vi "Controls to Commands 2016.vi"(10 "Pilot-CoPilot Controls":T3) -> (2 "Robot Commands":T1)   [LabVIEW 2015]
uses:
  Robot Control Outputs 2016.ctl
  Robot Commands 2016.ctl
  Load SS/Roller State.ctl
  Global Variables/Temp Variables.vi
  Global Variables/Settings.vi
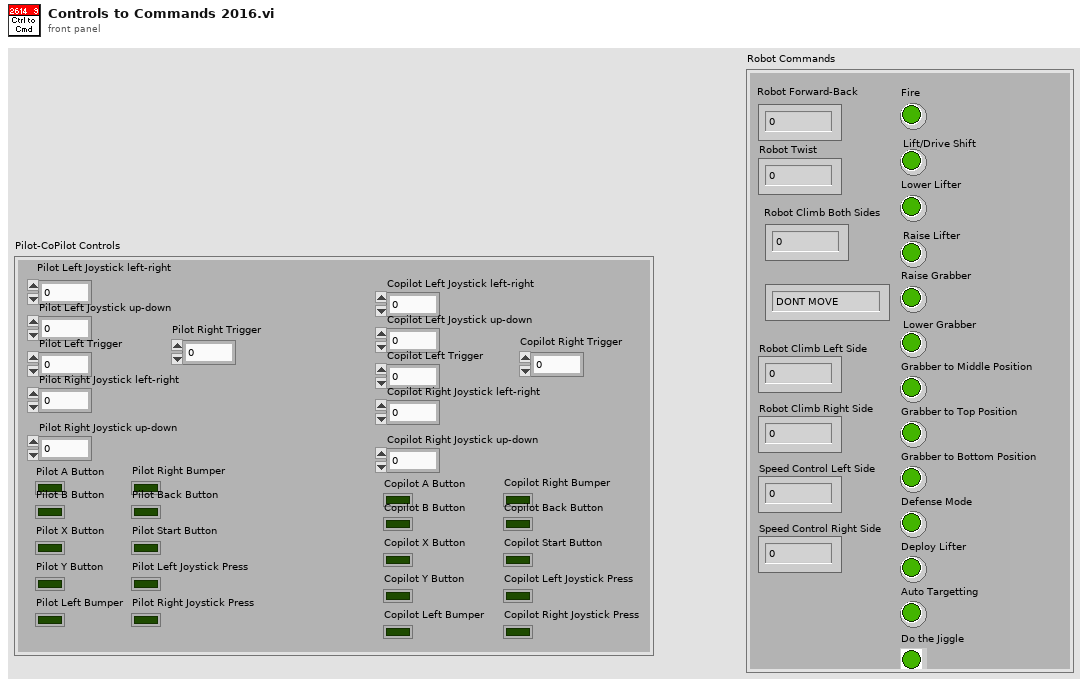
[diagram p1: front panel]
types:
  T1 = typedef "Robot Commands 2016.ctl" = cluster{"Robot Forward-Back":dbl, "Robot Twist":dbl, "Fire":bool, "Lift/Drive Shift":bool, "Raise Lifter":bool, "Raise Grabber":bool, "Lower Grabber":bool, "Roller":T2, "Robot Climb Both Sides":dbl, "Grabber to Middle Position":bool, "Grabber to Top Position":bool, "Grabber to Bottom Position":bool, "Robot Climb Left Side":dbl, "Robot Climb Right Side":dbl, "Speed Control Left Side":dbl, "Speed Control Right Side":dbl, "Lower Lifter":bool, "Defense Mode":bool, "Deploy Lifter":bool, "Auto Targetting":bool, "Do the Jiggle":bool}
  T2 = typedef "Roller State.ctl" = enum16{"DONT MOVE", "Intake", "Outtake"}
  T3 = typedef "Robot Control Outputs 2016.ctl" = cluster{"Pilot Left Joystick left-right":dbl, "Pilot Left Joystick up-down":dbl, "Pilot A Button":bool, "Pilot B Button":bool, "Pilot X Button":bool, "Pilot Y Button":bool, "Pilot Left Bumper":bool, "Pilot Right Bumper":bool, "Pilot Back Button":bool, "Pilot Start Button":bool, "Pilot Left Joystick Press":bool, "Pilot Right Joystick Press":bool, "Pilot Left Trigger":dbl, "Pilot Right Joystick left-right":dbl, "Pilot Right Joystick up-down":dbl, "Pilot Right Trigger":dbl, "Copilot Left Joystick left-right":dbl, "Copilot Left Joystick up-down":dbl, "Copilot A Button":bool, "Copilot B Button":bool, "Copilot X Button":bool, "Copilot Y Button":bool, "Copilot Left Bumper":bool, "Copilot Right Bumper":bool, "Copilot Back Button":bool, "Copilot Start Button":bool, "Copilot Left Joystick Press":bool, "Copilot Right Joystick Press":bool, "Copilot Left Trigger":dbl, "Copilot Right Joystick left-right":dbl, "Copilot Right Joystick up-down":dbl, "Copilot Right Trigger":dbl}
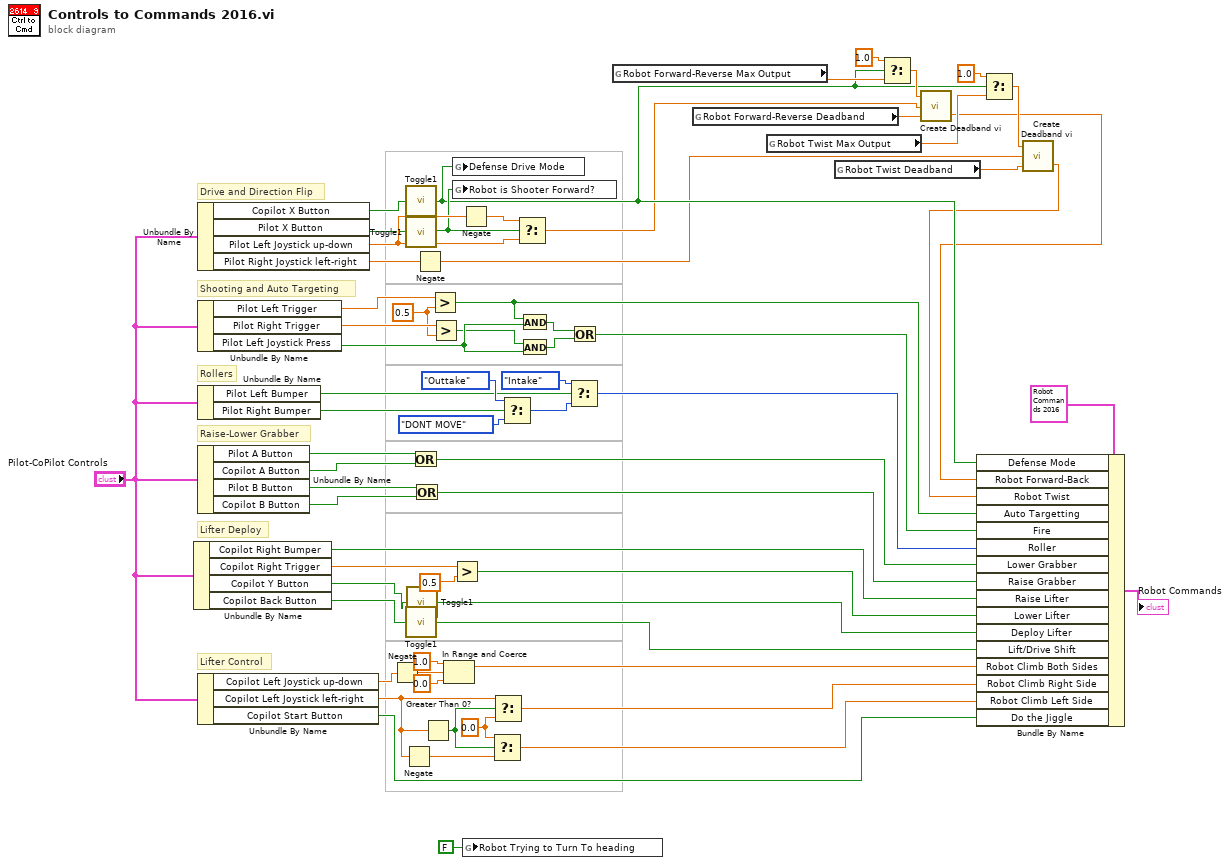
[diagram p0: block diagram]
diagram:
  w28 = 0.0 ("t")
  w63 = 0.5 ("y")
  # "Lifter Control"
  # "Lifter Deploy"
  # "Raise-Lower Grabber"
  # "Rollers"
  # "Shooting and Auto Targeting"
  # "Drive and Direction Flip"
  n1 = Unbundle By Name("Pilot-CoPilot Controls") -> ("Copilot Right Bumper"=w34:bool, "Copilot Right Trigger"=w32:dbl, "Copilot Y Button"=w17:bool, "Copilot Back Button"=w22:bool)
  n2 = Unbundle By Name("Pilot-CoPilot Controls") -> ("Copilot X Button"=w21:bool, "Pilot X Button"=w46:bool, "Pilot Left Joystick up-down"=w48:dbl, "Pilot Right Joystick left-right"=w49:dbl)
  n3 = Unbundle By Name("Pilot-CoPilot Controls") -> ("Pilot Left Trigger"=w64:dbl, "Pilot Right Trigger"=w65:dbl, "Pilot Left Joystick Press"=w61:bool)
  n4 = Unbundle By Name("Pilot-CoPilot Controls") -> ("Pilot Left Bumper"=w52:bool, "Pilot Right Bumper"=w51:bool)
  n5 = Unbundle By Name("Pilot-CoPilot Controls") -> ("Pilot A Button"=w44:bool, "Copilot A Button"=w43:bool, "Pilot B Button"=w42:bool, "Copilot B Button"=w41:bool)
  n6 = Unbundle By Name("Pilot-CoPilot Controls") -> ("Copilot Left Joystick up-down"=w30:dbl, "Copilot Left Joystick left-right"=w25:dbl, "Copilot Start Button"=w15:bool)
  n7 = Negate(x=w30) -> (-x=w35:dbl)
  n8 = Negate(x=w25) -> (-x=w26:dbl)
  n9 = call "Toggle1.vi"("Boolean"=w21) -> ("Driver Switch 2"=w6:bool)
  n10 = call "Toggle1.vi"("Boolean"=w46) -> ("Driver Switch 2"=w45:bool)
  n11 = call "Toggle1.vi"("Boolean"=w22) -> ("Driver Switch 2"=w18:bool)
  n12 = call "Toggle1.vi"("Boolean"=w17) -> ("Driver Switch 2"=w16:bool)
  n13 = Or(x=w44, y=w43) -> (x .or. y?=w40:bool)
  n14 = Or(x=w42, y=w41) -> (x .or. y?=w39:bool)
  n15 = Negate(x=w49) -> (-x=w4:dbl)
  n16 = Greater Than 0?(x=w25) -> (x > 0?=w27:bool)
  n17 = Greater?(x=w64, y=w63) -> (0:w62:bool)
  n18 = Greater?(x=w65, y=w63) -> (0:w60:bool)
  n19 = In Range and Coerce(upper limit=1.0 ("lower limit"), x=w35, lower limit=0.0) -> (coerced(x)=w29:dbl)  [unwired: 1 out]
  n20 = Greater?(x=w32, y=0.5) -> (0:w31:bool)
  n21 = global write "Temp Variables.vi" "Defense Drive Mode"(w6) -> ()
  n22 = global write "Temp Variables.vi" "Robot is Shooter Forward?"(w45) -> ()
  n23 = Negate(x=w48) -> (-x=w47:dbl)
  n24 = global write "Temp Variables.vi" "Robot Trying to Turn To heading"(FALSE ("Robot Trying to Turn To heading")) -> ()
  n25 = Select(t=w28, s=w27, f=w26) -> (s? t:f=w23:dbl)
  n26 = Select(t=w25, s=w27, f=w28) -> (s? t:f=w24:dbl)
  n27 = Select(t=Roller_State."Outtake" ("Roller State"), s=w51, f=Roller_State."DONT MOVE" ("Roller State")) -> (s? t:f=w56:T2)
  n28 = Select(t=w47, s=w45, f=w48) -> (s? t:f=w5:dbl)
  n29 = And(x=w62, y=w61) -> (x .and. y?=w58:bool)
  n30 = And(x=w60, y=w61) -> (x .and. y?=w59:bool)
  n31 = Select(t=Roller_State."Intake" ("Roller State"), s=w52, f=w56) -> (s? t:f=w50:T2)
  n32 = Or(x=w58, y=w59) -> (x .or. y?=w57:bool)
  n33 = global read "Settings.vi" "Robot Forward-Reverse Max Output"() -> (w11:dbl)
  n34 = global read "Settings.vi" "Robot Forward-Reverse Deadband"() -> (w13:dbl)
  n35 = global read "Settings.vi" "Robot Twist Max Output"() -> (w8:dbl)
  n36 = global read "Settings.vi" "Robot Twist Deadband"() -> (w14:dbl)
  n37 = Select(t=1.0, s=w6, f=w11) -> (s? t:f=w12:dbl)
  n38 = call "Create Deadband vi.vi"("Input Deadband"=w13, "Input"=w5, "Output Upper Limit"=w12) -> ("Output"=w3:dbl)  [unwired: 1 in]
  n39 = Select(t=1.0, s=w6, f=w8) -> (s? t:f=w9:dbl)
  n40 = call "Create Deadband vi.vi"("Input Deadband"=w14, "Input"=w4, "Output Upper Limit"=w9) -> ("Output"=w2:dbl)  [unwired: 1 in]
  n41 = Bundle By Name(cluster=T1 {"Robot Forward-Back"=0.0, "Robot Twist"=0.0, "Fire"=FALSE, "Lift/Drive Shift"=FALSE, "Raise Lifter"=FALSE, "Raise Grabber"=FALSE, "Lower Grabber"=FALSE, "Roller"=enum."DONT MOVE", "Robot Climb Both Sides"=0.0, "Grabber to Middle Position"=FALSE, "Grabber to Top Position"=FALSE, "Grabber to Bottom Position"=FALSE, "Robot Climb Left Side"=0.0, "Robot Climb Right Side"=0.0, "Speed Control Left Side"=0.0, "Speed Control Right Side"=0.0, "Lower Lifter"=FALSE, "Defense Mode"=FALSE, "Deploy Lifter"=FALSE, "Auto Targetting"=FALSE, "Do the Jiggle"=FALSE} ("Robot Commands"), "Defense Mode"=w6, "Robot Forward-Back"=w3, "Robot Twist"=w2, "Auto Targetting"=w62, "Fire"=w57, "Roller"=w50, "Lower Grabber"=w40, "Raise Grabber"=w39, "Raise Lifter"=w34, "Lower Lifter"=w31, "Deploy Lifter"=w16, "Lift/Drive Shift"=w18, "Robot Climb Both Sides"=w29, "Robot Climb Right Side"=w24, "Robot Climb Left Side"=w23, "Do the Jiggle"=w15) -> (→"Robot Commands":T1)
